vi "Flatten Value.vi"(8 "Error In":errorcluster, 11 "Path In":refnum<class "Path.lvclass">) -> (0 "Error Out":errorcluster, 1 "Value":string, 3 "Path Out":refnum<class "Path.lvclass">)   [LabVIEW 2017, in "Tree API.lvlib" / "Path.lvclass"]
uses:
  Path.lvclass
  Tree Manager/Tree.lvclass
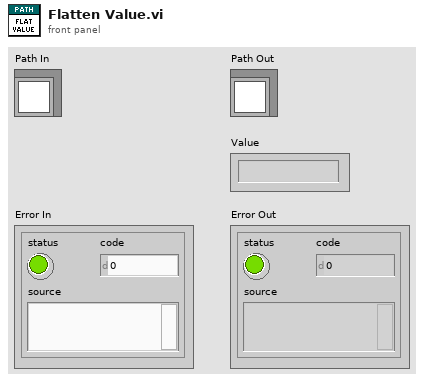
[diagram p1: front panel]
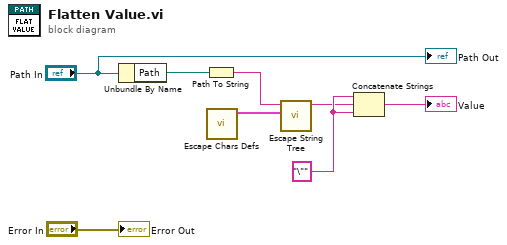
[diagram p0: block diagram]
diagram:
  w5 = "\"" ("string")
  n1 = Unbundle By Name("Path In") -> ("Path"=w8:path)
  n2 = Path To String(path=w8) -> (string=w4:string)
  n3 = call "Escape Chars Defs.vi"() -> ("Escapes"=w3:cluster{"String":string, "Escape":string}[])  [unwired: 11 in]
  n4 = call "Escape String Tree.vi"("Escapes"=w3, "String In"=w4) -> ("String Out"=w2:string)  [unwired: 9 in]
  n5 = Concatenate Strings(w5, w2, w5) -> (→"Value":string)
  "Path Out" <- "Path In"
  "Error Out" <- "Error In"
